vi "DragHandler.vi"(10 "Coords":T2, 11 "Type":T1) -> (1 "ValidDrag?":bool, 3 "IncDrag":cluster{"X Cen":dbl, "Y Cen":dbl})   [LabVIEW 2014]
uses:
  <vilib>/Utility/miscctls.llb/LVPoint32TypeDef.ctl
  <vilib>/event_ctls.llb/lveventtype.ctl
panel:
  out "Inc Drag X":i32
  out "Inc Drag Y":i32
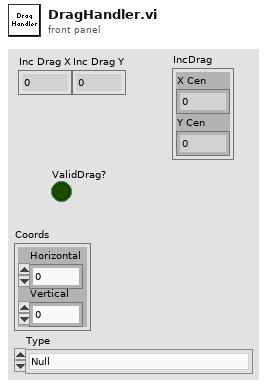
[diagram p1: front panel]
types:
  T1 = typedef "lveventtype.ctl" = enum32{"Null", "Timeout", "Annotation Menu Selection", "Annotation Menu Selection?", "App Instance Close", "App Instance Close?", "Autoscale Range Change", "Bookmark Info Change", "Cell Edit", "Cell Edit?", "Cursor Grab", "Cursor Grab?", "Cursor Menu Selection", "Cursor Menu Selection?", "Cursor Move", "Cursor Release", "Data Change", "Direction Change", "Display State Change", "Drag Ended", "Drag Enter", "Drag Leave", "Drag Over", "Drag Source Update", "Drag Starting", "Drag Starting?", "Drop", "Exec State Change", "Key Down", "Key Down?", "Key Repeat", "Key Repeat?", "Key Up", "Listbox Double Click", "Menu Activation?", "Menu Selection (App)", "Menu Selection? (App)", "Menu Selection (User)", "Mouse Down", "Mouse Down?", "Mouse Enter", "Mouse Leave", "Mouse Move", "Mouse Up", "Mouse Wheel", "NI Security User Change (App)", "Pane Size", "Panel Close", "Panel Close?", "Panel Resize", "Plot Attribute Change", "Scale Range Change", "Shortcut Menu Activation?", "Shortcut Menu Selection (App)", "Shortcut Menu Selection? (App)", "Shortcut Menu Selection (User)", "Tree Double Click", "Tree Drag", "Tree Drag?", "Tree Drop", "Tree Drop?", "Tree Item Close", "Tree Item Close?", "Tree Item Open", "Tree Item Open?", "User Event", "Value Change"}
  T2 = typedef "LVPoint32TypeDef.ctl" = cluster{"Horizontal":i32, "Vertical":i32}
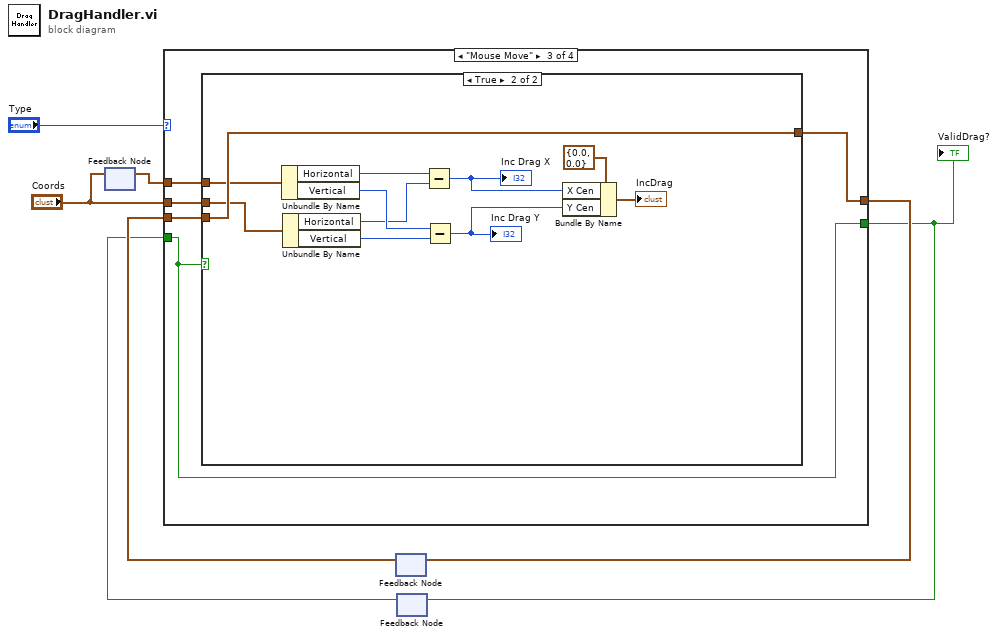
[diagram p0: block diagram]
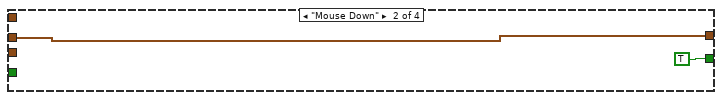
[diagram p3: hidden frame]
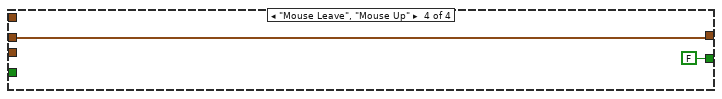
[diagram p5: hidden frame]
diagram:
  n1 = feedback #1() -> (w1:T2)  [unwired: 1 in]
  n2 = feedback-in #1("Coords") -> ()
  n3 = feedback #2() -> (w6:T2)  [unwired: 1 in]
  n4 = feedback #3() -> (w4:bool)  [unwired: 1 in]
  n5 = case shown="\"Mouse Move\"" "Type" {
    tunnel: [w9 w10 w14 w29] -> w7
    tunnel: "Coords" -> [_ w10 w16 w29]
    tunnel: w6 -> [w9 _ w15 _]
    tunnel: [w8 TRUE w13 FALSE] -> w5
    tunnel: w4 -> [w8 _ w13 _]
    tunnel: w1 -> [_ _ w12 _]
    frame "Null", Default {
    }
    frame "Mouse Down" {
    }
    frame "Mouse Move" {
      n6 = case shown="True" w13 {
        tunnel: w16 -> [_ w18]
        tunnel: w15 -> [w17 w28]
        tunnel: [w17 w28] -> w14
        tunnel: w12 -> [_ w23]
        frame False {
        }
        frame True {
          n7 = Unbundle By Name(w23) -> ("Horizontal"=w26:i32, "Vertical"=w27:i32)
          n8 = Unbundle By Name(w18) -> ("Horizontal"=w24:i32, "Vertical"=w25:i32)
          n9 = Subtract(x=w26, y=w24) -> (x-y=w22:i32)
          "Inc Drag X" <- w22
          n10 = Subtract(x=w27, y=w25) -> (x-y=w21:i32)
          "Inc Drag Y" <- w21
          n11 = Bundle By Name(cluster=cluster{"X Cen":dbl, "Y Cen":dbl} {"X Cen"=0.0, "Y Cen"=0.0} ("OffSet"), "X Cen"=w22, "Y Cen"=w21) -> (→"IncDrag":cluster{"X Cen":dbl, "Y Cen":dbl})
        }
      }
    }
    frame "Mouse Leave", "Mouse Up" {
    }
  }
  "ValidDrag?" <- w5
  n12 = feedback-in #2(w7) -> ()
  n13 = feedback-in #3(w5) -> ()
